vi "GlobalVariables_DIALMain.vi"() -> ()   [LabVIEW 2014]
uses:
  NCARLabviewTesting/TypeDefinitions.llb/TypeDef_MainControlSystem.ctl
panel:
  in  "Tab Control":enum32{"Main Globals", "Laser Globals"}(tab)
  out "ChildAbort":bool
  in  "VI Timeout":dbl=5.0
  in  "Global File Paths":path[](array[path])=[path "/Freundlein/Users/Bobby/Desktop/NCARLabviewTesting/SingleControls/Log_SetUserComment.vi", path "/Freundlein/Users/Bobby/Desktop/NCARLabviewTesting/SingleControls/Idle_Password.vi"]
  out "RunAsChild":bool
  out "GlobalStop":bool
  in  "PermissionLevel":i32
  out "Children Details":T2(array[cluster]) {"MainControlSystems" items=["Counting System Control", "Counting System Display", "Laser Control", "Laser Locking", "Weather Station", "Data Display"]}
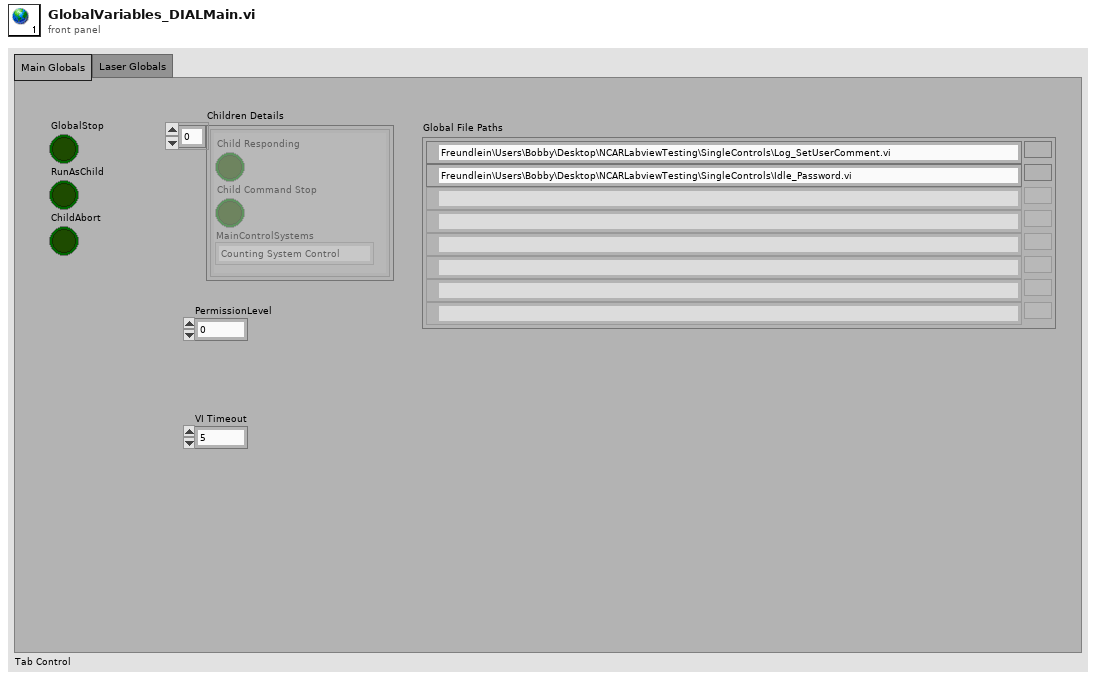
[diagram p1: front panel]
types:
  T1 = typedef "TypeDef_MainControlSystem.ctl" = u16
  T2 = cluster{"Child Command Stop":bool, "Child Responding":bool, "MainControlSystems":T1}[]
diagram:
